vi "USRP Dummy DMA to Memory (Host).vi"() -> ()   [LabVIEW 2016]
uses:
  <vilib>/userdefined/High Color/nirio_resource_hc.ctl
  <vilib>/FPGAPlugInAG/USRP 294xR; 295xR 200 MSps/niLvFpga_Open_USRP 294xR; 295xR 200 MSps.vi
  <vilib>/rvi/interface/common/dynamic/niFpgaDynamicAddResources.vi
  <vilib>/FPGAPlugInAG/Dynamic/niLvFpga_Download_Dynamic.vi
  <vilib>/FPGAPlugInAG/Dynamic/niLvFpga_Run_Dynamic.vi
  <vilib>/Utility/error.llb/Error Cluster From Error Code.vi
  <vilib>/rvi/errors/niLvFpgaAdjustHostInterfaceError.vi
  <vilib>/rvi/interface/common/niFpgaWaitOnOcc.vi
  <vilib>/FPGAPlugInAG/Dynamic/niLvFpga_Close_Dynamic.vi
  <vilib>/rvi/interface/nirviOpenFPGA/nirviOpenFPGA.xnode
  Bitfiles/USRP-RIO-Streami_DummyDMA_USRPDummy(FPGA)_kay5ptBR-r4.lvbitx
  <vilib>/rvi/interface/nirviMethod/nirviMethod.xnode
  <vilib>/rvi/interface/nirviReadWriteControl/nirviReadWriteControl.xnode
  <vilib>/rvi/interface/nirviCloseFPGA/nirviCloseFPGA.xnode
  <vilib>/rvi/errors/niLvFpgaMergeErrorWithErrorCode.vi
  <vilib>/rvi/interface/Simulation/niFpgaSimulationCallBeginRW.vi
  <instrlib>/niUsrpRio/Config/v1/Host/niUsrpRio Config v1 Host.lvlib
  NiFpgaLv.dll
  <vilib>/FPGAPlugInAG/Dynamic/niLvFpga_StopFifo_Dynamic.vi
  <vilib>/FPGAPlugInAG/Dynamic/niLvFpga_ConfigureFifo_Dynamic.vi
  <vilib>/FPGAPlugInAG/Dynamic/niLvFpga_StartFifo_Dynamic.vi
  <vilib>/FPGAPlugInAG/Dynamic/niLvFpga_ReadFifo_Dynamic.vi
panel:
  in  "Fixed Fetch?":bool=TRUE
  out "Random Number":u64 format="%016x"
  in  "Decimate (200MHz)":u32=2
  out "Host Transfer Slider":u64(slide) scale=0.0..68719476736.0
  in  "Flush FIFO?":bool
  out "Control Loop":i32
  in  "Host FIFO Fetch":u32=131072
  in  "Reset Host Count?":bool
  in  "Stop Transfer?":bool
  in  "Reset FPGA Count?":bool
  out "FPGA Side FIFO":cluster{u32, u32}(slide)={66, 63} scale=0.0..2047.0
  out "Host Side FIFO":cluster{u32, u32}(slide) scale=0.0..67108863.0
  out "Data Loop":i32
  out "Fetch Loop":i32
  out "Host Count":u64
  in  "Number of Samples":u64=68719476736
  out "FPGA Count":u64
  in  "Start Transfer":bool
  in  "terminate":bool
  out "Elements Remaining":u32
  out "Data":u64[](array[numeric]) format="%016x"
  out "Timeout Counts":u64
  in  "Reset Timeouts?":bool
  out "Actual Depth":u32
  in  "Host Requested Depth":u32=67108864
  out "error out":errorcluster
  in  "Resource Name":T1="PXI2Slot18Port1Dev1"
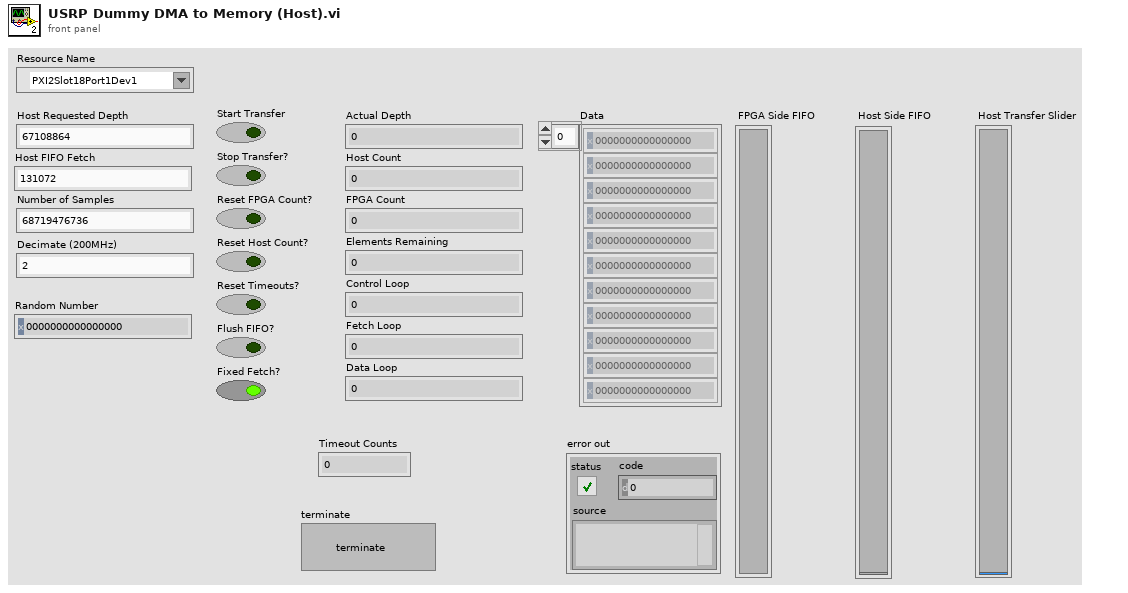
[diagram p1: front panel]
types:
  T1 = typedef "nirio_resource_hc.ctl" = tag
  T2 = typedef "niUsrpRio Config v1 Host.lvlib/niUsrpRio Session.ctl" = cluster{"FPGA Interface":refnum<k20>, "RIO Interface Number":u32, "Data Clock Rate":u32, "FPGA Data Clock Rate":u32, "Global Settings Register Bus":T3, "Radio 0 Settings Register Bus":T3, "Radio 1 Settings Register Bus":T3, "Radio Settings Bus Semaphore":T4, "DB Queues":T5[], "Characterization Data Valid?":bool, "EEPROM Header":T6, "Device Data Header":T7, "EEPROM Characterization Header":T8, "Characterization Data":T9[], "FPGA Current Version":u32, "FPGA Oldest Compatible Version":u32, "Fixed Logic Current Version":u32, "Fixed Logic Oldest Compatible Version":u32, "FPGA Radio Settings Bus Current Version":u32, "FPGA Radio Settings Bus Oldest Compatible Version":u32, "FPGA Board Config Current Version":u32, "FPGA Board Config Oldest Compatible Version":u32, "Daughterboard Clock Rate":u32, "daughterboard configuration session handles":u64[]}
  T3 = typedef "niInstr Register Bus v0 Host.lvlib/Register Bus Session.ctl" = refnum<queue>
  T4 = typedef "Semaphore RefNum" = refnum<k1>
  T5 = typedef "niUsrpRio Config v1 Host.lvlib/DB Queue Reference.ctl" = refnum<queue>
  T6 = typedef "niUsrpRio Config v1 Host.lvlib/EEPROM Header.ctl" = cluster{"Checksum":u32, "Product Code":u16, "Hardware Current Version":u16, "Hardware Oldest Compatible Version":u16, "EEPROM Map Current Version":u16, "EEPROM Map Oldest Compatible Version":u16, "User Password":string, "Pointer to Factory Header":u32, "Pointer to User Header":u32, "Recommended Interval":u16, "Number of Reserved Bytes":i32, "Number of Daughterboards":u8, "Daughterboard IDs":u16[], "Daughterboard Serial Numbers":string[]}
  T7 = typedef "niUsrpRio Config v1 Host.lvlib/EEPROM Device Data Header.ctl" = cluster{"Checksum":u32, "Number of Channels":u8, "Number of Gain Settings":u16[], "Pointer to Characterization Data":u32[], "Number of Reserved Bytes":i32, "Number of Frequencies":u16[]}
  T8 = typedef "niUsrpRio Config v1 Host.lvlib/EEPROM Characterization Header.ctl" = cluster{"Checksum":u32, "Date":timestamp, "Temperature":sgl, "Misc. Info":string, "Pointer to Device Data Header":u32, "Number of Reserved Bytes":i32}
  T9 = typedef "niUsrpRio Config v1 Host.lvlib/Characterization Data.ctl" = cluster{"Gains[dB]":dbl[], "Frequencies [Hz]":dbl[], "IQ Imbalance Table":T10[], "Measured Gains[dB]":dbl[][]}
  T10 = typedef "niUsrpRio Config v1 Host.lvlib/IQ Imbalance.ctl" = cluster{"Gain Imbalance [linear]":dbl, "Phase Imbalance [radians]":dbl, "Offset":cdb}
  T11 = cluster{"Maximum Amount Used":u32, "Current Amount Used":u32}
  T12 = cluster{"Running Max":u32, "Elements Remaining":u32}
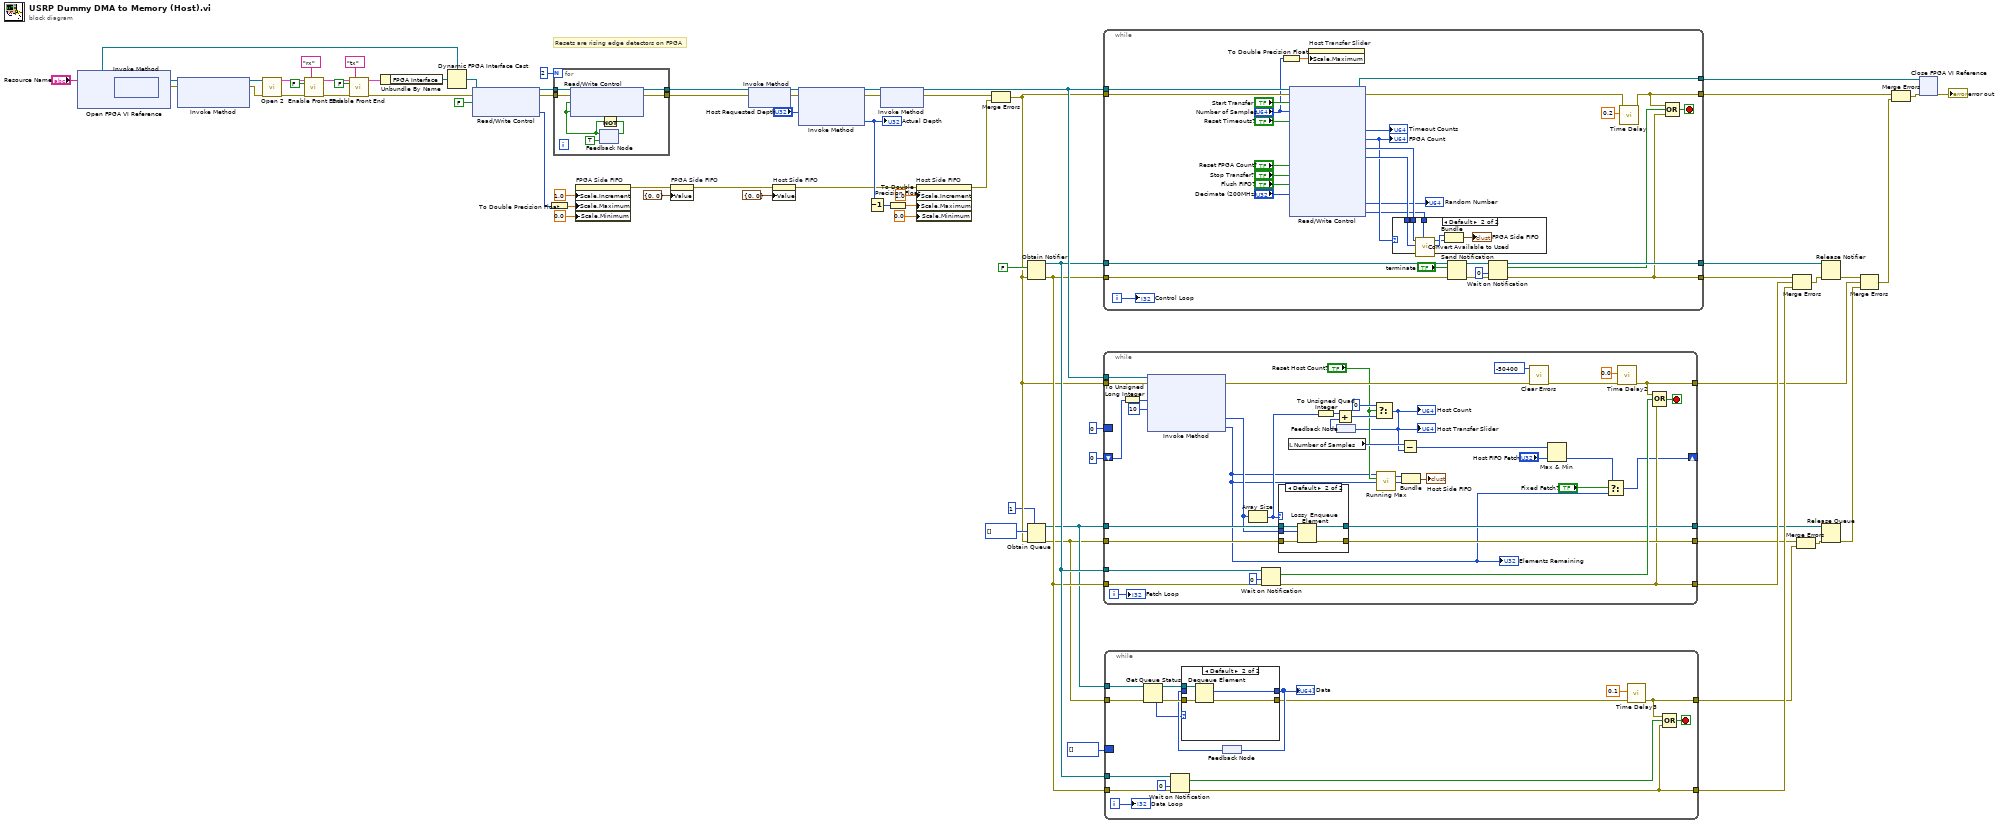
[diagram p0: block diagram]
diagram:
  # "Resets are rising edge detectors on FPGA"
  n1 = xnode "Open FPGA VI Reference"("resource name"="Resource Name") -> ("FPGA VI Reference Out"=w7:refnum<k20>, "error out"=w6:errorcluster)  [unwired: 1 in]
  n2 = xnode "Invoke Method"("FPGA VI Reference In"=w7, "error in"=w6) -> ("FPGA VI Reference Out"=w5:refnum<k20>, "error out"=w4:errorcluster)
  n3 = xnode "Invoke Method"("FPGA VI Reference In"=w5, "error in"=w4) -> ("FPGA VI Reference Out"=w3:refnum<k20>, "error out"=w2:errorcluster)  [unwired: 1 in]
  n4 = call <instrlib>:"Open 2.vi"("fpga ref"=w3, "error in"=w2) -> ("niUsrpRio Session (out)"=w64:T2, "error out"=w69:errorcluster)  [unwired: 12 in]
  n5 = call <instrlib>:"Enable Front End.vi"("niUsrpRio Session"=w64, "scope"="rx", "enable"=FALSE, "error in"=w69) -> ("niUsrpRio Session (out)"=w65:T2, "error out"=w68:errorcluster)  [unwired: 10 in]
  n6 = call <instrlib>:"Enable Front End.vi"("niUsrpRio Session"=w65, "scope"="tx", "enable"=FALSE, "error in"=w68) -> ("niUsrpRio Session (out)"=w61:T2, "error out"=w60:errorcluster)  [unwired: 10 in]
  n7 = Unbundle By Name(w61) -> ("FPGA Interface"=w59:refnum<k20>)
  n8 = Dynamic FPGA Interface Cast(Session In=w7, Type=w59) -> (Session Out=w58:refnum<k20>)
  n9 = xnode "Read/Write Control"("FPGA VI Reference In"=w58, "error in"=w60, "Start Transfer?"=FALSE ("send data?")) -> ("FPGA VI Reference Out"=w36:refnum<k20>, "error out"=w35:errorcluster, "FPGA FIFO Depth"=w21:u32)
  n10 = To Double Precision Float(number=w21) -> (double precision float=w23:dbl)
  n11 = for {
    N: 2 -> [_]
    tunnel: w36 -> [w82]
    tunnel: w35 -> [w81]
    tunnel: [w80] -> w34
    tunnel: [w79] -> w33
    n12 = feedback #1(TRUE) -> (w77:bool)
    n13 = xnode "Read/Write Control"("FPGA VI Reference In"=w82, "error in"=w81, "Reset Timeouts?"=w77, "Reset FPGA Count?"=w77) -> ("FPGA VI Reference Out"=w80:refnum<k20>, "error out"=w79:errorcluster)
    n14 = Not(x=w77) -> (.not. x?=w76:bool)
    n15 = feedback-in #1(w76) -> ()
  }
  n16 = property on="FPGA Side FIFO" class="Slide (strict)"("Scale.Increment"=1.0 ("Scale.Range:Increment"), "Scale.Maximum"=w23, "Scale.Minimum"=0.0 ("Scale.Range:Minimum")) -> (error out=w16:errorcluster)  [unwired: 2 in, 1 out]
  n17 = property on="FPGA Side FIFO" class="Slide (strict)"(error in=w16, "Value"=cluster{u32, u32} {0, 0} ("FPGA Side FIFO")) -> (error out=w19:errorcluster)  [unwired: 1 in, 1 out]
  n18 = xnode "Invoke Method"("FPGA VI Reference In"=w34, "error in"=w33) -> ("FPGA VI Reference Out"=w75:refnum<k20>, "error out"=w74:errorcluster)
  n19 = property on="Host Side FIFO" class="Slide (strict)"(error in=w19, "Value"=cluster{u32, u32} {0, 0} ("FPGA Side FIFO")) -> (error out=w15:errorcluster)  [unwired: 1 in, 1 out]
  n20 = xnode "Invoke Method"("FPGA VI Reference In"=w75, "error in"=w74, "Requested Depth"="Host Requested Depth") -> ("FPGA VI Reference Out"=w71:refnum<k20>, "error out"=w72:errorcluster, "Actual Depth"=w20:u32)
  "Actual Depth" <- w20
  n21 = Decrement(x=w20) -> (x-1=w26:u32)
  n22 = xnode "Invoke Method"("FPGA VI Reference In"=w71, "error in"=w72) -> ("FPGA VI Reference Out"=w56:refnum<k20>, "error out"=w22:errorcluster)
  n23 = To Double Precision Float(number=w26) -> (double precision float=w8:dbl)
  n24 = property on="Host Side FIFO" class="Slide (strict)"(error in=w15, "Scale.Increment"=1.0 ("Data Entry Limits:Increment"), "Scale.Maximum"=w8, "Scale.Minimum"=0.0 ("Data Entry Limits:Minimum")) -> (error out=w13:errorcluster)  [unwired: 1 in, 1 out]
  n25 = Merge Errors(w22, w13) -> (w14:errorcluster)
  n26 = Obtain Notifier(notification data type=FALSE, error in (no error)=w14) -> (notifier out=w48:refnum<notifier>, error out=w47:errorcluster)  [unwired: 2 in, 1 out]
  n27 = Obtain Queue(max queue size (-1, unlimited)=1, element data type=u64[] [] ("Data"), error in (no error)=w14) -> (queue out=w40:refnum<queue>, error out=w39:errorcluster)  [unwired: 2 in, 1 out]
  n28 = while {
    tunnel: w56 -> [w113]
    tunnel: w14 -> [w112]
    tunnel: w48 -> [w109]
    tunnel: w47 -> [w108]
    tunnel: [w103] -> w53
    tunnel: [w96] -> w52
    tunnel: [w98] -> w31
    tunnel: [w97] -> w30
    i -> [w89]
    stop <- w102 stop-if-true
    n29 = To Double Precision Float(number="Number of Samples") -> (double precision float=w86:dbl)
    n30 = xnode "Read/Write Control"("FPGA VI Reference In"=w113, "error in"=w112, "Start Transfer?"="Start Transfer", "Number of Samples"="Number of Samples", "Reset Timeouts?"="Reset Timeouts?", "Reset FPGA Count?"="Reset FPGA Count?", "Stop Transfer?"="Stop Transfer?", "Flush FIFO?"="Flush FIFO?", "Decimate (200MHz)"="Decimate (200MHz)") -> ("FPGA VI Reference Out"=w97:refnum<k20>, "error out"=w111:errorcluster, "Timeout Count"=→"Timeout Counts":u64, "FPGA Count"=w90:u64, "Space Available"=w95:u32, "Min Space Available"=w93:u32, "Random Number"=→"Random Number":u64, "FPGA FIFO Depth"=w83:u32)
    "FPGA Count" <- w90
    n31 = property on="Host Transfer Slider" class="Slide (strict)"("Scale.Maximum"=w86) -> ()  [unwired: 2 in, 2 out]
    n32 = case shown="Default" w90 {
      tunnel: w83 -> [_ w119]
      tunnel: w95 -> [_ w118]
      tunnel: w93 -> [_ w117]
      frame 0 {
      }
      frame Default {
        n33 = call "Convert Available to Used.vi"("Size"=w119, "Minimum Amount Available"=w117, "Current Amount Available"=w118) -> ("Maximum Amount Used"=w116:u32, "Current Amount Used"=w115:u32)  [unwired: 5 in]
        n34 = Bundle("Maximum Amount Used"=w116, "Current Amount Used"=w115) -> (→"FPGA Side FIFO":T11)  [unwired: 1 in]
      }
    }
    n35 = Send Notification(notification="terminate", notifier=w109, error in (no error)=w108) -> (notifier out=w105:refnum<notifier>, error out=w104:errorcluster)
    n36 = Wait on Notification(notifier=w105, timeout in ms (-1)=0, error in (no error)=w104) -> (notifier out=w103:refnum<notifier>, notification=w101:bool, error out=w96:errorcluster)  [unwired: 1 in, 1 out]
    n37 = call "Time Delay"("error in (no error)"=w111, "Delay Time (s)"=0.2) -> ("error out"=w98:errorcluster)  [unwired: 9 in]
    n38 = Compound Arithmetic op=OR(w98, w101, w96) -> (w102:bool)
    "Control Loop" <- w89
  }
  n39 = while {
    tunnel: [w152] -> w32
    tunnel: w56 -> [w155]
    tunnel: w14 -> [w154]
    border: u64 0 -> [_]
    tunnel: w48 -> [w148]
    tunnel: w47 -> [w147]
    tunnel: [w138] -> w50
    tunnel: [w143] -> w44
    tunnel: w40 -> [w144]
    tunnel: w39 -> [w142]
    tunnel: [w141] -> w43
    shift-right: [w124] -> _
    shift-left: u64 0 -> [w132]
    i -> [w145]
    stop <- w150 stop-if-true
    n40 = To Unsigned Long Integer(number=w132) -> (unsigned 32bit integer=w131:u32)
    n41 = xnode "Invoke Method"("FPGA VI Reference In"=w155, "error in"=w154, "Number of Elements"=w131, "Timeout (ms)"=10) -> ("error out"=w140:errorcluster, "Data"=w139:u64[], "Elements Remaining"=w123:u32)  [unwired: 1 out]
    "Elements Remaining" <- w123
    n42 = Array Size(array=w139) -> (size(s)=w135:i32)
    n43 = Wait on Notification(notifier=w148, timeout in ms (-1)=0, error in (no error)=w147) -> (notification=w146:bool, error out=w138:errorcluster)  [unwired: 1 in, 2 out]
    n44 = case shown="Default" w135 {
      tunnel: w144 -> [w159 w164]
      tunnel: [w159 w163] -> w143
      tunnel: w142 -> [w158 w162]
      tunnel: [w158 w161] -> w141
      tunnel: w139 -> [_ w160]
      frame 0 {
      }
      frame Default {
        n45 = Lossy Enqueue Element(queue=w164, element=w160, error in (no error)=w162) -> (queue out=w163:refnum<queue>, error out=w161:errorcluster)  [unwired: 2 out]
      }
    }
    n46 = local read "Number of Samples"() -> (w134:u64)
    n47 = To Unsigned Quad Integer(1:w135) -> (0:w157:u64)
    n48 = feedback #2() -> (w156:u64)
    n49 = Add(x=w157, y=w156) -> (x+y=w137:u64)
    n50 = Select(t=u64 0, s="Reset Host Count?", f=w137) -> (s? t:f=w122:u64)
    "Host Count" <- w122
    "Host Transfer Slider" <- w122
    n51 = feedback-in #2(w122) -> ()
    n52 = call "Running Max.vi"("Reset"="Reset Host Count?", "Next Value"=w123) -> ("Running Max"=w128:u32)  [unwired: 5 in]
    n53 = Subtract(x=w134, y=w122) -> (x-y=w133:u64)
    n54 = Bundle("Running Max"=w128, "Elements Remaining"=w123) -> (→"Host Side FIFO":T12)  [unwired: 1 in]
    n55 = call <vilib>:"Clear Errors.vi"("error in (no error)"=w140, "specific error code to clear (0: all)"=-50400) -> ("error out"=w130:errorcluster)  [unwired: 4 in, 1 out]
    n56 = Max & Min(x=w133, y="Host FIFO Fetch") -> (min(x,y)=w120:u64)  [unwired: 1 out]
    n57 = Select(t=w120, s="Fixed Fetch?", f=w123) -> (s? t:f=w124:u64)
    n58 = call "Time Delay2"("error in (no error)"=w130, "Delay Time (s)"=0.0) -> ("error out"=w152:errorcluster)  [unwired: 9 in]
    n59 = Compound Arithmetic op=OR(w152, w146, w138) -> (w150:bool)
    "Fetch Loop" <- w145
  }
  n60 = while {
    tunnel: w48 -> [w179]
    tunnel: w47 -> [w178]
    tunnel: [w165] -> w46
    tunnel: w40 -> [w176]
    tunnel: w39 -> [w175]
    tunnel: [w167] -> w38
    border: u64[] [] -> [_]
    i -> [w181]
    stop <- w169 stop-if-true
    n61 = Get Queue Status(queue=w176, error in (no error)=w175) -> (queue out=w173:refnum<queue>, error out=w174:errorcluster, # elements in queue=w170:i32)  [unwired: 1 in, 5 out]
    n62 = Wait on Notification(notifier=w179, timeout in ms (-1)=0, error in (no error)=w178) -> (notification=w177:bool, error out=w165:errorcluster)  [unwired: 1 in, 2 out]
    n63 = feedback #3() -> (w172:u64[])
    n64 = case shown="Default" w170 {
      tunnel: [w183 w187] -> w168
      tunnel: [w182 w184] -> w171
      tunnel: w174 -> [w183 w186]
      tunnel: w173 -> [_ w185]
      tunnel: w172 -> [w182 _]
      frame 0 {
      }
      frame Default {
        n65 = Dequeue Element(queue=w185, error in (no error)=w186) -> (element=w184:u64[], error out=w187:errorcluster)  [unwired: 1 in, 2 out]
      }
    }
    "Data" <- w171
    n66 = feedback-in #3(w171) -> ()
    n67 = call "Time Delay3"("error in (no error)"=w168, "Delay Time (s)"=0.1) -> ("error out"=w167:errorcluster)  [unwired: 9 in]
    n68 = Compound Arithmetic op=OR(w167, w177, w165) -> (w169:bool)
    "Data Loop" <- w181
  }
  n69 = Merge Errors(w52, w50, w46) -> (w51:errorcluster)
  n70 = Merge Errors(w43, w38) -> (w42:errorcluster)
  n71 = Release Notifier(notifier=w53, error in (no error)=w51) -> (error out=w49:errorcluster)  [unwired: 1 in, 2 out]
  n72 = Release Queue(queue=w44, error in (no error)=w42) -> (error out=w41:errorcluster)  [unwired: 1 in, 2 out]
  n73 = Merge Errors(w49, w32, w41) -> (w9:errorcluster)
  n74 = Merge Errors(w31, w9) -> (w10:errorcluster)
  n75 = xnode "Close FPGA VI Reference"("FPGA VI Reference In"=w30, "error in"=w10) -> ("error out"=→"error out":errorcluster)
